vi "link -- read rusout file.vi"(6 "# of peaks to show":i32, 8 "rus out file path":path=path "C:/Data/GloveBox/Pu/rprcyl") -> (0 "freqs":dbl[](array[numeric]), 3 "rusout out":T1, 5 "size(s)":i32)   [LabVIEW 2014]
uses:
  link -- rusout.ctl
  <vilib>/Utility/file.llb/Read From Spreadsheet File (string).vi
panel:
  in  "rusout dummy":T1
  in  "Color Box":u32(colorbox)
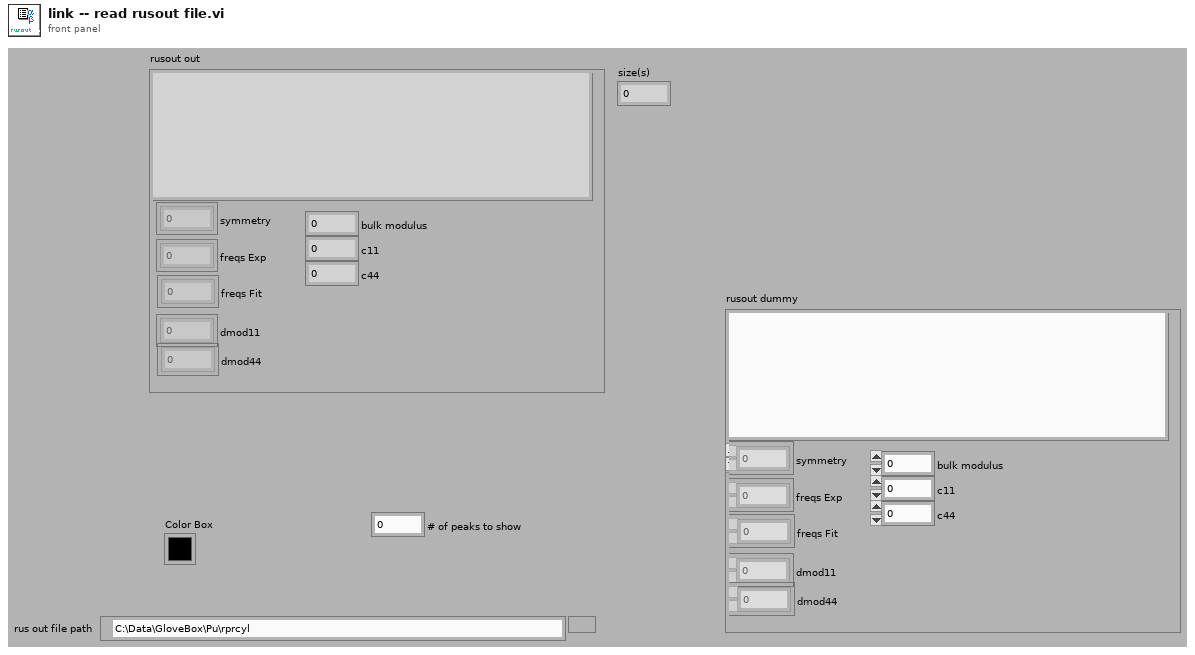
[diagram p1: front panel]
types:
  T1 = typedef "link -- rusout.ctl" = cluster{"freqs Exp":dbl[], "symmetry":i32[], "dmod11":dbl[], "dmod44":dbl[], "freqs Fit":dbl[], "header":string, "bulk modulus":dbl, "c11":dbl, "c44":dbl}
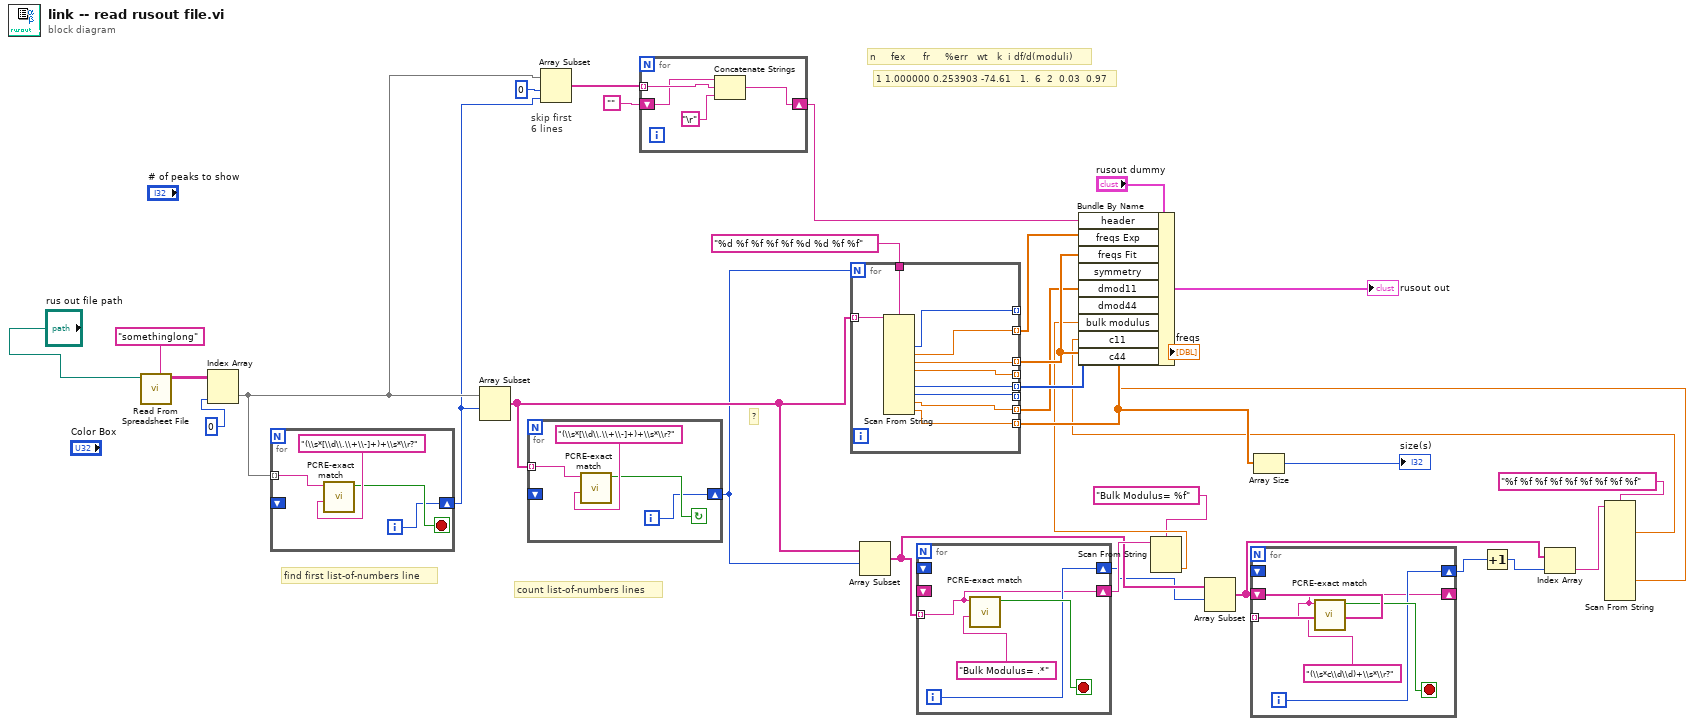
[diagram p0: block diagram]
diagram:
  # "count list-of-numbers lines"
  # "find first list-of-numbers line"
  # "skip first \n6 lines"
  # "?"
  # "1 1.000000 0.253903 -74.61   1.  6  2  0.03  0.97"
  # "n     fex      fr     %err   wt   k  i df/d(moduli)"
  n1 = call-poly <vilib>:"Read From Spreadsheet File.vi"("delimiter (\\t)"="somethinglong" ("delimiter (\\t)"), "file path (dialog if empty)"="rus out file path") -> ("all rows"=w31:string[][])  [unwired: 5 in, 4 out]
  n2 = Index Array(array=w31, index (col)=0 ("index (row)")) -> (element=w2:string[])  [unwired: 1 in]
  n3 = for {
    tunnel: w2 -> [w37] mode=indexing
    shift-right: [w34] -> w1
    shift-left: _ -> [_]
    i -> [w34]
    stop <- w35 stop-if-true
    n4 = call "PCRE-exact match.vi"("regular expression"="(\\s*[\\d\\.\\+\\-]+)+\\s*\\r?" ("format string"), "input string"=w37) -> ("exact match"=w35:bool)  [unwired: 8 in, 1 out]
  }
  n5 = Array Subset(array=w2, index=w1) -> (w16:string[])  [unwired: 1 in]
  n6 = for {
    tunnel: w16 -> [w41] mode=indexing
    shift-right: [w38] -> w15
    shift-left: _ -> [_]
    i -> [w38]
    stop <- w39 continue-if-true
    n7 = call "PCRE-exact match.vi"("regular expression"="(\\s*[\\d\\.\\+\\-]+)+\\s*\\r?" ("format string"), "input string"=w41) -> ("exact match"=w39:bool)  [unwired: 8 in, 1 out]
  }
  n8 = Array Subset(array=w2, index=0 ("index (row)"), length=w1) -> (w22:string[])
  n9 = for {
    tunnel: w22 -> [w45] mode=indexing
    shift-right: [w42] -> w20
    shift-left: "" -> [w43]
    n10 = Concatenate Strings(w43, w45, "\r") -> (w42:string)
  }
  n11 = for {
    N: w15 -> [_]
    tunnel: w16 -> [w46] mode=indexing
    tunnel: [w55] -> _ mode=indexing
    tunnel: [w54] -> w19 mode=indexing
    tunnel: [w53] -> w27 mode=indexing
    tunnel: "%d %f %f %f %f %d %d %f %f" ("format string") -> [w47]
    tunnel: [w52] -> _ mode=indexing
    tunnel: [w51] -> w26 mode=indexing
    tunnel: [w50] -> _ mode=indexing
    tunnel: [w49] -> w25 mode=indexing
    tunnel: [w48] -> w18 mode=indexing
    n12 = Scan From String(format string=w47, input string=w46) -> (output 1=w55:i32, output 2=w54:dbl, output 3=w53:dbl, output 4=w52:dbl, output 6=w51:i32, output 7=w50:i32, output 8=w49:dbl, output 9=w48:dbl)  [unwired: 12 in, 3 out]
  }
  "freqs" <- w27
  n13 = Array Subset(array=w16, index=w15) -> (w12:string[])  [unwired: 1 in]
  n14 = for {
    tunnel: w12 -> [w56] mode=indexing
    shift-right: [w57] -> w11
    shift-left: _ -> [_]
    shift-right: [w56] -> w14
    shift-left: _ -> [_]
    i -> [w57]
    stop <- w58 stop-if-true
    n15 = call "PCRE-exact match.vi"("regular expression"="Bulk Modulus= .*" ("format string"), "input string"=w56) -> ("exact match"=w58:bool)  [unwired: 8 in, 1 out]
  }
  n16 = Scan From String(format string="Bulk Modulus= %f", input string=w14) -> (output 1=w13:dbl)  [unwired: 3 in, 3 out]
  n17 = Array Subset(array=w12, index=w11) -> (w8:string[])  [unwired: 1 in]
  n18 = for {
    tunnel: w8 -> [w60] mode=indexing
    shift-right: [w61] -> w10
    shift-left: _ -> [_]
    shift-right: [w60] -> _
    shift-left: _ -> [_]
    i -> [w61]
    stop <- w62 stop-if-true
    n19 = call "PCRE-exact match.vi"("regular expression"="(\\s*c\\d\\d)+\\s*\\r?" ("format string"), "input string"=w60) -> ("exact match"=w62:bool)  [unwired: 8 in, 1 out]
  }
  n20 = Array Size(array=w18) -> (size(s)=→"size(s)":i32)
  n21 = Increment(x=w10) -> (x+1=w9:i32)
  n22 = Index Array(array=w8, index=w9) -> (element=w7:string)
  n23 = Scan From String(format string="%f %f %f %f %f %f %f %f %f", input string=w7) -> (output 1=w5:dbl, output 7=w4:dbl)  [unwired: 18 in, 3 out]
  n24 = Bundle By Name(cluster="rusout dummy", "header"=w20, "freqs Exp"=w19, "freqs Fit"=w27, "symmetry"=w26, "dmod11"=w25, "dmod44"=w18, "bulk modulus"=w13, "c11"=w5, "c44"=w4) -> (→"rusout out":T1)
